vi "Telnet.vi"() -> ()   [LabVIEW 2013]
uses:
  <vilib>/addons/internet/NI_InternetTK_Core_VIs.lvlib
panel:
  out "error out":errorcluster
  out "data out":string
  in  "error in (no error)":errorcluster
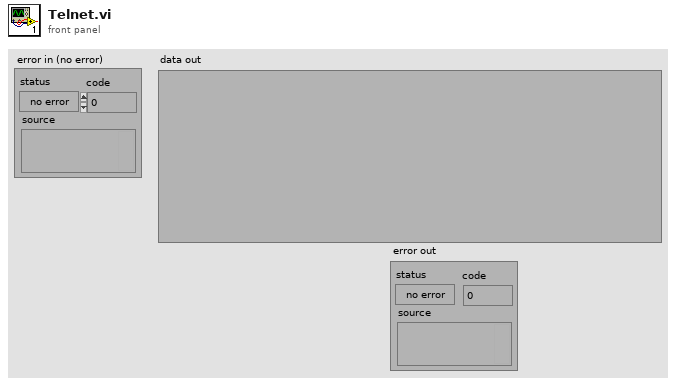
[diagram p1: front panel]
types:
  T1 = typedef "Telnet Session.ctl" = refnum<k1>
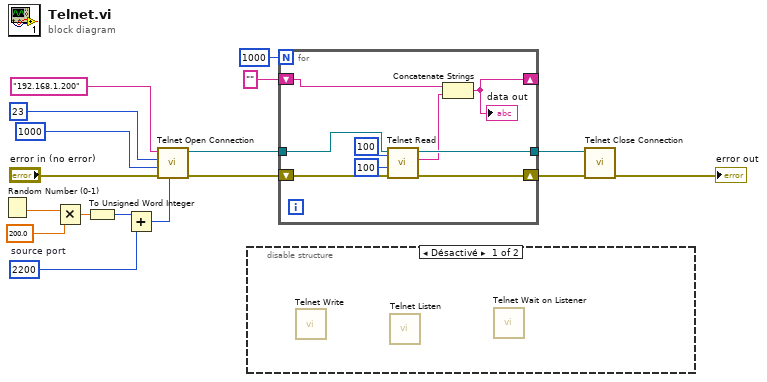
[diagram p0: block diagram]
diagram:
  w9 = u16 2200  # source port
  n1 = Random Number (0-1)() -> (number: 0 to 1=w11:dbl)
  n2 = Multiply(x=w11, y=200.0) -> (x*y=w13:dbl)
  n3 = To Unsigned Word Integer(number=w13) -> (unsigned 16bit integer=w10:u16)
  n4 = Add(x=w10, y=w9) -> (x+y=w8:u16)
  n5 = call <vilib>:"Telnet Open Connection.vi"("local port"=w8, "error in (no error)"="error in (no error)", "timeout ms (60000)"=1000, "remote port (23)"=u16 23, "address"="192.168.1.200") -> ("error out"=w6:errorcluster, "telnet connection"=w7:T1)  [unwired: 5 in]
  n6 = disable-structure shown="Désactivé" {
    frame Disabled {
      n7 = call <vilib>:"Telnet Write.vi"() -> ()  [unwired: 7 in, 3 out]
      n8 = call <vilib>:"Telnet Listen.vi"() -> ()  [unwired: 8 in, 4 out]
      n9 = call <vilib>:"Telnet Wait on Listener.vi"() -> ()  [unwired: 7 in, 5 out]
    }
    frame Enabled {
    }
  }
  n10 = for {
    N: 1000 -> [_]
    tunnel: w7 -> [w26]
    tunnel: [w22] -> w2
    shift-right: [w18] -> _
    shift-left: "" ("Chaîne") -> [w20]
    shift-right: [w21] -> w1
    shift-left: w6 -> [w25]
    n11 = call <vilib>:"Telnet Read.vi"("error in (no error)"=w25, "timeout ms (25000)"=100, "bytes to read"=100, "telnet connection"=w26) -> ("error out"=w21:errorcluster, "data out"=w19:string, "telnet connection out"=w22:T1)  [unwired: 3 in]
    n12 = Concatenate Strings(w20, w19) -> (w18:string)
    "data out" <- w18
  }
  n13 = call <vilib>:"Telnet Close Connection.vi"("error in (no error)"=w1, "telnet connection"=w2) -> ("error out"=→"error out":errorcluster)  [unwired: 8 in, 1 out]
